vi "Colorcycle2004.vi"   [LabVIEW 2013]
uses:
  <vilib>/Heliosphere Research LLC/Advanced Plotting Toolkit/api_plotting/LineProperties.ctl
  <vilib>/Heliosphere Research LLC/Advanced Plotting Toolkit/properties/Line.ctl
  <vilib>/Heliosphere Research LLC/Advanced Plotting Toolkit/properties/Line_Style.ctl
  <vilib>/Heliosphere Research LLC/Advanced Plotting Toolkit/typedefs/PlotColor.ctl
  <vilib>/Heliosphere Research LLC/Advanced Plotting Toolkit/properties/Marker.ctl
  <vilib>/Heliosphere Research LLC/Advanced Plotting Toolkit/properties/Marker_Style.ctl
  <vilib>/Heliosphere Research LLC/Advanced Plotting Toolkit/properties/Display.ctl
  <vilib>/Heliosphere Research LLC/Advanced Plotting Toolkit/Advanced Plotting Toolkit.lvlib
types:
  T1 = typedef "Advanced Plotting Toolkit.lvlib/LineProperties.ctl" = cluster{"Line":T2, "Marker":T5, "Display":T7}
  T2 = typedef "Advanced Plotting Toolkit.lvlib/Line.ctl" = cluster{"Style":T3, "Color":T4, "Width":sgl}
  T3 = typedef "Advanced Plotting Toolkit.lvlib/Line_Style.ctl" = enum16{"Automatic", "Solid", "Dashed", "Dotted", "Dash-dot", "Invisible"}
  T4 = typedef "Advanced Plotting Toolkit.lvlib/PlotColor.ctl" = u32
  T5 = typedef "Advanced Plotting Toolkit.lvlib/Marker.ctl" = cluster{"Style":T6, "Color":T4, "Size":dbl}
  T6 = typedef "Advanced Plotting Toolkit.lvlib/Marker_Style.ctl" = enum16{"Automatic", "Circle", "Square", "Triangle", "Diamond", "Star", "Invisible"}
  T7 = typedef "Advanced Plotting Toolkit.lvlib/Display.ctl" = cluster{"Alpha":dbl, "Z Order":dbl}
  T8 = typedef "Advanced Plotting Toolkit.lvlib/PlotID.ctl" = i32
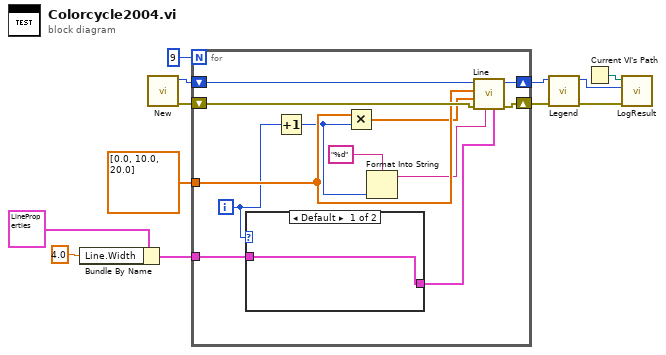
[diagram p0: block diagram]
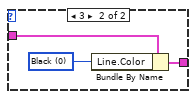
[diagram p2: hidden frame]
diagram:
  n1 = Bundle By Name(cluster=T1 {"Line"={"Style"=enum."Automatic", "Color"=2147483647, "Width"=nan}, "Marker"={"Style"=enum."Automatic", "Color"=2147483647, "Size"=nan}, "Display"={"Alpha"=nan, "Z Order"=nan}} ("Line Plot Properties"), "Line.Width"=sgl 4.0) -> (w2:T1)
  n2 = call <vilib>:"New.vi"() -> ("error out"=w9:errorcluster, "Plot ID"=w11:T8)  [unwired: 10 in]
  n3 = for {
    N: 9 -> [_]
    shift-right: [w21] -> w8
    shift-left: w11 -> [w24]
    tunnel: dbl[] [0.0, 10.0, 20.0] -> [w20]
    shift-right: [w22] -> w6
    shift-left: w9 -> [w23]
    tunnel: w2 -> [w14]
    i -> [w15]
    n4 = case shown="Default" w15 {
      tunnel: w14 -> [w25 w28]
      tunnel: [w25 w27] -> w13
      frame Default {
      }
      frame 3 {
        w26 = T4 0 items=["Automatic"=2147483647, "Black"=0, "White"=16777215, "Red"=16711680, "Green"=2263842, "Blue"=255, "Cyan"=65535, "Magenta"=16711935, "Yellow"=16776960] ("Line.Color")
        n5 = Bundle By Name(cluster=w28, "Line.Color"=w26) -> (w27:T1)
      }
    }
    n6 = Increment(x=w15) -> (x+1=w17:i32)
    n7 = Multiply(x=w20, y=w17) -> (x*y=w19:dbl[])
    n8 = Format Into String(format string="%d", w17) -> (resulting string=w16:string)  [unwired: 2 in, 1 out]
    n9 = call <vilib>:"Line.vi"("Properties"=w13, "Legend Title"=w16, "error in (no error)"=w23, "Y Data"=w19, "X Data"=w20, "Plot ID"=w24) -> ("error out"=w22:errorcluster, "Plot ID out"=w21:T8)  [unwired: 4 in]
  }
  n10 = call <vilib>:"Legend.vi"("error in (no error)"=w6, "Plot ID"=w8) -> ("error out"=w5:errorcluster, "Plot ID Out"=w7:T8)  [unwired: 8 in]
  n11 = Current VI's Path() -> (path=w12:path)
  n12 = call "LogResult.vi"("Test Result"=w5, "Test Artifact"=w7, "VI Path"=w12) -> ()  [unwired: 9 in]
